vi "method.vi"(8 "error in (no error)":errorcluster, 11 "class 1 in":refnum<class "class 1.lvclass">) -> (0 "error out":errorcluster, 3 "class 1 out":refnum<class "class 1.lvclass">)   [LabVIEW 2023, in "class 1.lvclass"]
uses:
  class 1.lvclass
  class 1.lvclass/class 1.ctl
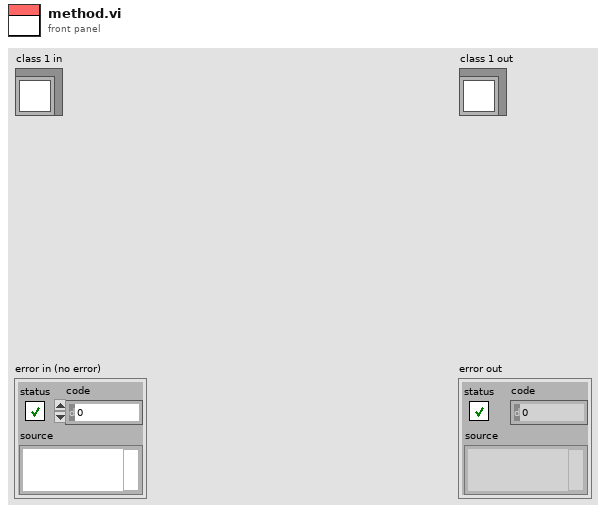
[diagram p1: front panel]
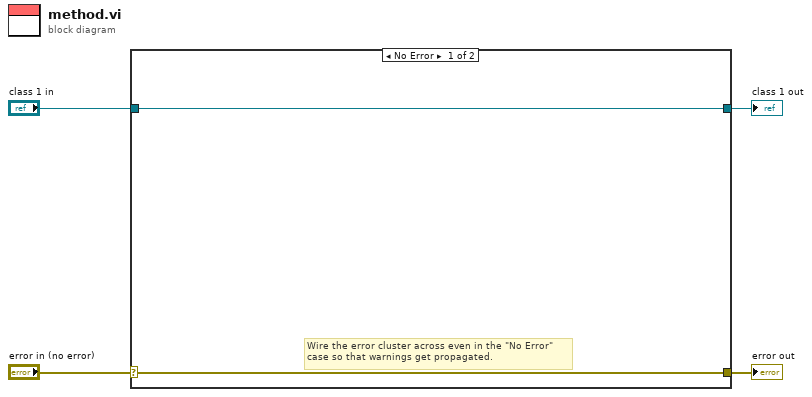
[diagram p0: block diagram]
diagram:
  n1 = case shown="No Error" "error in (no error)" {
    selector: "error in (no error)" -> [w5 w8]
    tunnel: [w5 w8] -> w3
    tunnel: [w6 w7] -> w1
    tunnel: "class 1 in" -> [w6 w7]
    frame No Error {
      # "Wire the error cluster across even in the \"No Error\"\ncase so that warnings get propagated."
    }
    frame Error {
    }
  }
  "error out" <- w3
  "class 1 out" <- w1
